vi "Read Instr.vi"(8 "error in (no error)":errorcluster, 11 "PIPXI40 Base in":refnum<class "PIPX40 Base.lvclass">) -> (0 "error out":errorcluster, 2 "Instrument handle":refnum<visa-resource-name>, 3 "PIPXI40 Base out":refnum<class "PIPX40 Base.lvclass">)   [LabVIEW 2020, in "Pickering.lvlib" / "PIPX40 Base.lvclass"]
uses:
  PIPX40 Base.lvclass
  PIPX40 Base.lvclass/PIPX40 Base.ctl
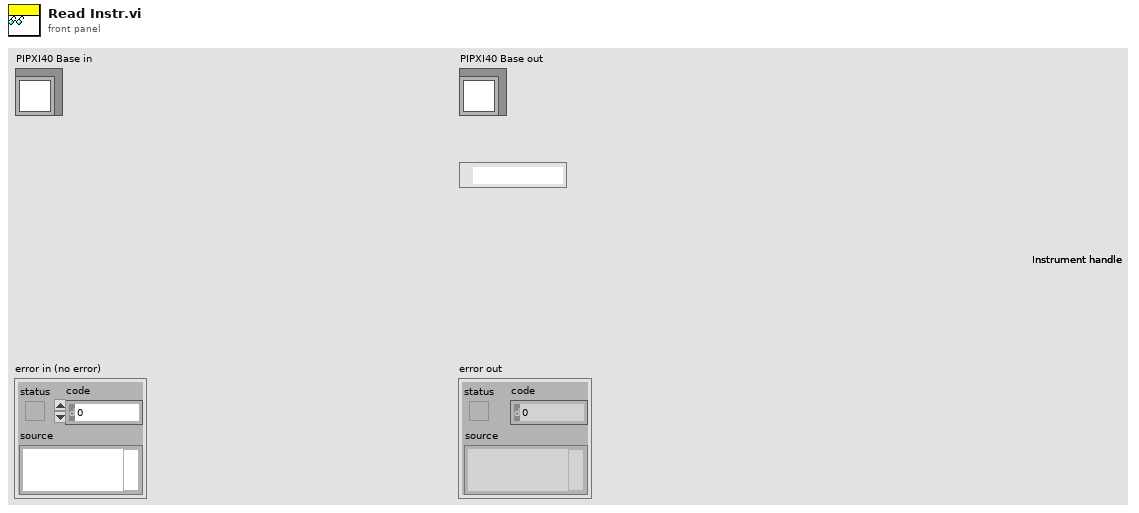
[diagram p1: front panel]
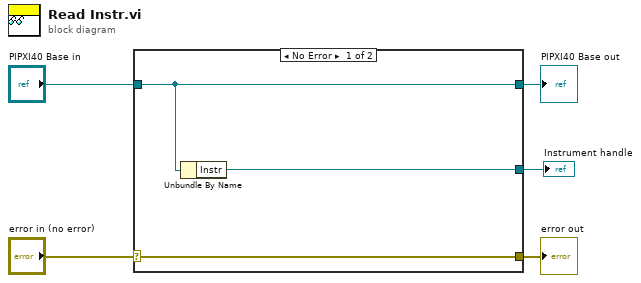
[diagram p0: block diagram]
diagram:
  n1 = case shown="No Error" "error in (no error)" {
    selector: "error in (no error)" -> [w8 w9]
    tunnel: [w8 w9] -> w4
    tunnel: [w7 w10] -> w2
    tunnel: "PIPXI40 Base in" -> [w7 w10]
    tunnel: [w6 _] -> w1
    frame No Error {
      n2 = Unbundle By Name(w7) -> ("Instr"=w6:refnum<visa-resource-name>)
    }
    frame Error {
    }
  }
  "error out" <- w4
  "PIPXI40 Base out" <- w2
  "Instrument handle" <- w1
